vi "PV ActiveLine - OffsetDisplay (TPG362).vi"(7 "W/R":bool, 8 "Fehler (Eingang)":errorcluster, 9 "Sensor 2 Set":dbl format="%.4e", 10 "Sensor 1 Set":dbl format="%.4e", 11 "Referenz in":refnum<visa-resource-name>) -> (0 "Cluster (Ausgang)":errorcluster, 1 "Sensor2 Get":dbl format="%.4e", 2 "Sensor 1 Get":dbl format="%.4e", 3 "Referenz out":refnum<visa-resource-name>)   [LabVIEW 2013, in "PV ActiveLine.lvlib"]
doc: "OFD - Offset Display (Linear Gauges)\n\nTransmit: OFD [,sa.aaaaEsaa,sb.bbbbEsbb]\nReceive: sa.aaaaEsaa,sb.bbbbEsbb\n\nsa.aaaaEsaa Gauge 1 Offset, [in current pressure unit] (default = 0.0000E+00)\nsa.aaaaEsaa Gauge 2 Offset, [in current pressure unit] (default = 0.0000E+00)\n\nValues can be entered in any format. They are internally converted into the floating point format."
uses:
  <instrlib>/PV ActiveLine/PV ActiveLine.lvlib
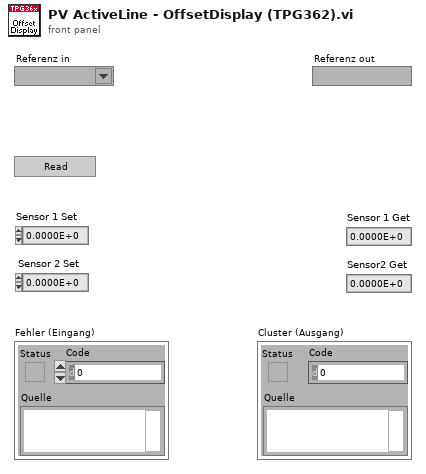
[diagram p1: front panel]
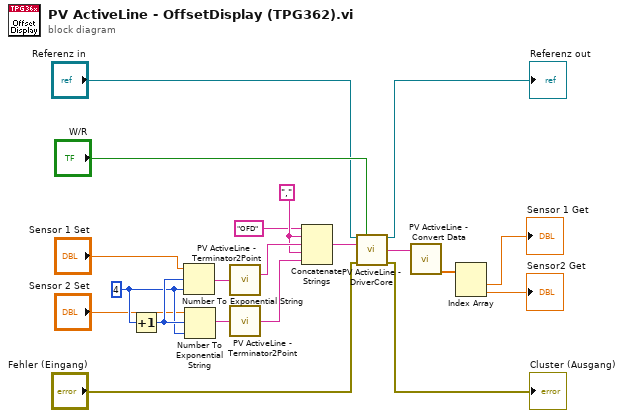
[diagram p0: block diagram]
diagram:
  w7 = ","
  w3 = u8 4 ("Kommastellen")
  n1 = Increment(x=w3) -> (x+1=w6:u8)
  n2 = Number To Exponential String(number="Sensor 1 Set", precision (6)=w3, 3:w6) -> (E-format string=w11:string)  [unwired: 1 in]
  n3 = Number To Exponential String(number="Sensor 2 Set", precision (6)=w3, 3:w6) -> (E-format string=w10:string)  [unwired: 1 in]
  n4 = call <instrlib>:"PV ActiveLine - Terminator2Point.vi"("Eingangstring"=w11) -> ("Ausgangstring"=w9:string)
  n5 = call <instrlib>:"PV ActiveLine - Terminator2Point.vi"("Eingangstring"=w10) -> ("Ausgangstring"=w8:string)
  n6 = Concatenate Strings("OFD" ("Command"), w7, w9, w7, w8) -> (w4:string)
  n7 = call <instrlib>:"PV ActiveLine - DriverCore.vi"("Referenz in"="Referenz in", "Write/Read"="W/R", "Command"=w4, "Fehler (Eingang)"="Fehler (Eingang)") -> ("Referenz out"=→"Referenz out":refnum<visa-resource-name>, "String Out"=w15:string, "Cluster (Ausgang)"=→"Cluster (Ausgang)":errorcluster)  [unwired: 9 in]
  n8 = call <instrlib>:"PV ActiveLine - Convert Data.vi"("String in"=w15) -> ("DBL out"=w14:dbl[])  [unwired: 7 in, 3 out]
  n9 = Index Array(array=w14) -> (element #1=→"Sensor 1 Get":dbl, element #2=→"Sensor2 Get":dbl)  [unwired: 2 in]
